vi "EPICS_test.vi"() -> ()   [LabVIEW 2015]
uses:
  Program Files (x86)/National Instruments/LabVIEW 2019/user.lib/caLab/Private/Put_I32_PV.vi
  Program Files (x86)/National Instruments/LabVIEW 2019/user.lib/caLab/Private/Put_I32-1D_PV-1D.vi
panel:
  in  "close":bool
  in  "stop":bool
  in  "start":bool
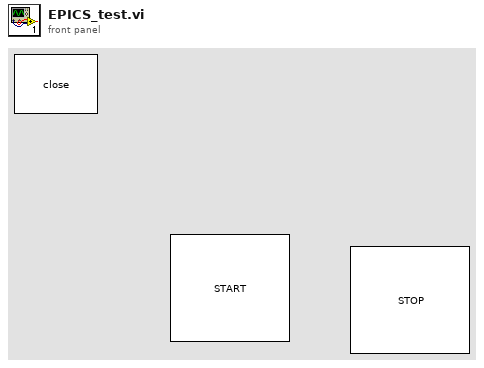
[diagram p1: front panel]
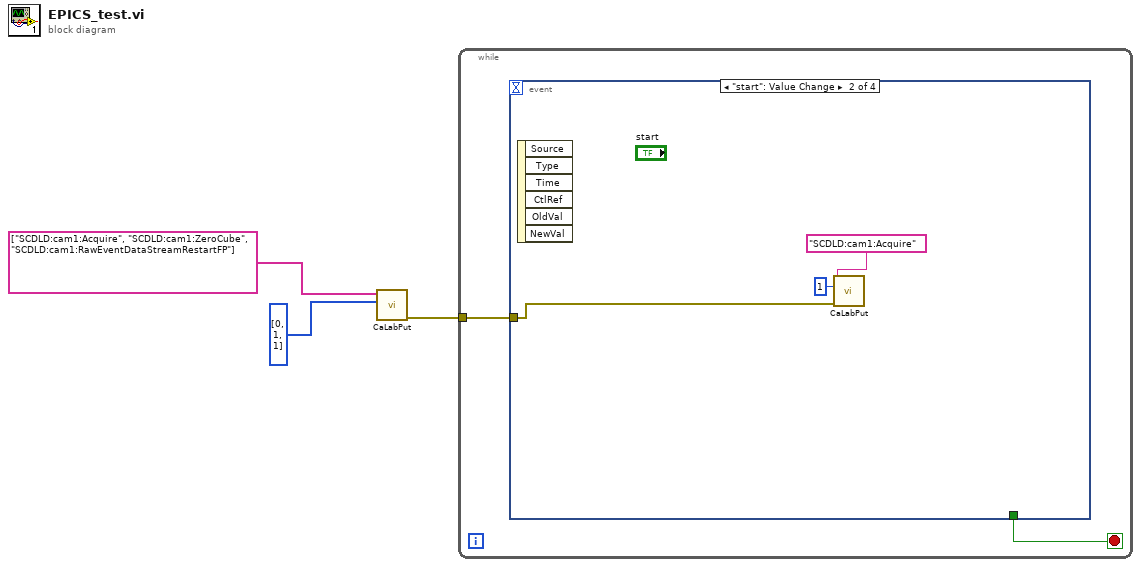
[diagram p0: block diagram]
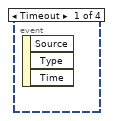
[diagram p2: hidden frame]
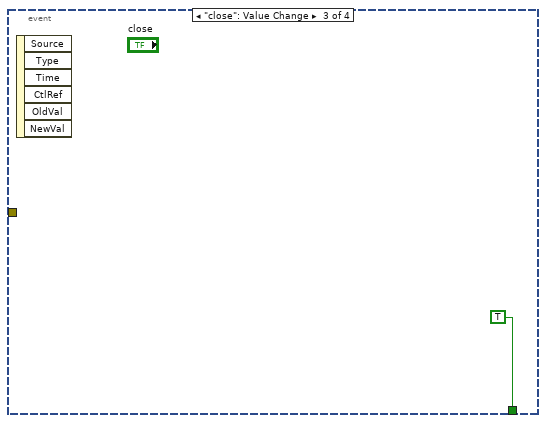
[diagram p3: hidden frame]
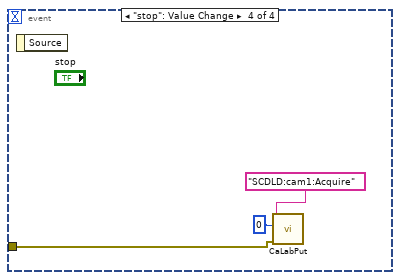
[diagram p4: hidden frame]
diagram:
  n1 = call-poly "CaLabPut.vi"("Values"=i32[] [0, 1, 1], "PV Names"=string[] ["SCDLD:cam1:Acquire", "SCDLD:cam1:ZeroCube", "SCDLD:cam1:RawEventDataStreamRestartFP"]) -> ("Error out"=w1:errorcluster)  [unwired: 6 in, 3 out]
  n2 = while {
    tunnel: w1 -> [w5]
    stop <- w4 stop-if-true
    n3 = event shown="[1] \"start\": Value Change" {
      selector: _ -> [_ _ _ _]
      dyn-events: _ -> [_ _ _ _]
      timeout: _ -> [_ _ _ _]
      tunnel: w5 -> [_ w6 _ w10]
      tunnel: [_ _ TRUE _] -> w4
      event Timeout {
        n4 = event-data() -> ()  [unwired: 1 in, 3 out]
      }
      event "start": Value Change {
        n5 = event-data() -> ()  [unwired: 1 in, 6 out]
        n6 = call-poly "CaLabPut.vi"("Error in (no error)"=w6, "Value"=1, "PV Name"="SCDLD:cam1:Acquire") -> ()  [unwired: 5 in, 4 out]
      }
      event "close": Value Change {
        n7 = event-data() -> ()  [unwired: 1 in, 6 out]
      }
      event "stop": Value Change {
        n8 = event-data() -> ()  [unwired: 1 in, 1 out]
        n9 = call-poly "CaLabPut.vi"("Error in (no error)"=w10, "Value"=0, "PV Name"="SCDLD:cam1:Acquire") -> ()  [unwired: 5 in, 4 out]
      }
    }
  }
